vi "Reorient DH Matrix.vi"(10 "z":dbl[](array[numeric]), 11 "Original Frame":T1) -> (3 "Reoriented Frame":T1)   [LabVIEW 2017, in "NI_Robotics_3DKinematics.lvlib"]
uses:
  <vilib>/robotics/Kinematics/Plotting/NI_Robotics_3DKinematics.lvlib
  <vilib>/Analysis/Matrix/Datatypes/RealMatrix.ctl
  <vilib>/Analysis/_algsub.llb/Real Vector Norm.vi
  <vilib>/Analysis/NI_AALPro.lvlib
  <vilib>/robotics/Kinematics/NI_Kinematics.lvlib
  <vilib>/Analysis/Matrix/NI_Matrix.lvlib
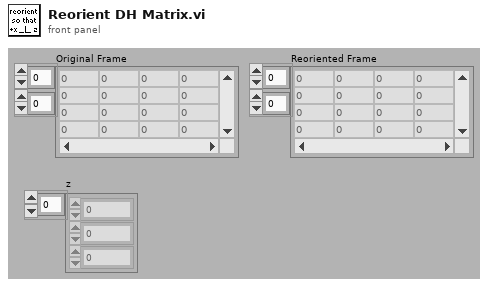
[diagram p1: front panel]
types:
  T1 = typedef "NI_Matrix.lvlib/RealMatrix.ctl" = dbl[][]
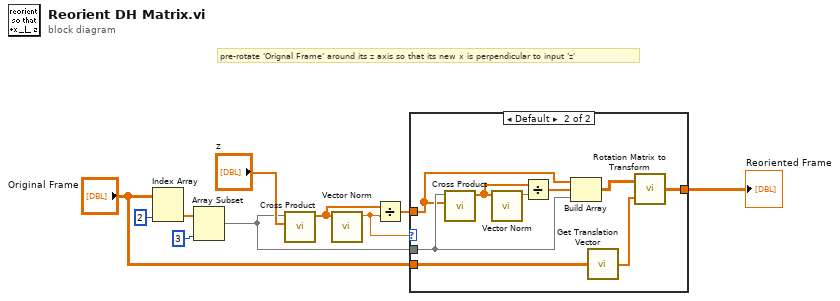
[diagram p0: block diagram]
diagram:
  # "pre-rotate 'Orignal Frame' around its z axis so that its new x is perpendicular to input 'z'"
  n1 = Index Array(array="Original Frame", index (col)=2 ("index (row)")) -> (element=w10:dbl[])  [unwired: 1 in]
  n2 = Array Subset(array=w10, length=3) -> (w1:dbl[])  [unwired: 1 in]
  n3 = call <vilib>:"Cross Product.vi"("B Vector"="z", "A Vector"=w1) -> ("Cross Product"=w4:dbl[])  [unwired: 8 in, 1 out]
  n4 = call-poly <vilib>:"Vector Norm.vi"("Input Vector"=w4) -> ("norm"=w5:dbl)  [unwired: 9 in, 1 out]
  n5 = Divide(x=w4, y=w5) -> (x/y=w6:dbl[])
  n6 = case shown="Default" w5 {
    tunnel: w6 -> [_ w14]
    tunnel: [w11 w15] -> w8
    tunnel: w1 -> [_ w16]
    tunnel: "Original Frame" -> [w11 w13]
    frame 0 {
    }
    frame Default {
      n7 = call <vilib>:"Cross Product.vi"("B Vector"=w14, "A Vector"=w16) -> ("Cross Product"=w19:dbl[])  [unwired: 8 in, 1 out]
      n8 = call-poly <vilib>:"Vector Norm.vi"("Input Vector"=w19) -> ("norm"=w20:dbl)  [unwired: 9 in, 1 out]
      n9 = Divide(x=w19, y=w20) -> (x/y=w18:dbl[])
      n10 = Build Array(w14, w18, w16) -> (w17:T1)
      n11 = call <vilib>:"Get Translation Vector.vi"("transform"=w13) -> ("translation vector"=w12:dbl[])
      n12 = call <vilib>:"Rotation Matrix to Transform.vi"("translation vector"=w12, "rotation matrix"=w17) -> ("transform"=w15:T1)
    }
  }
  "Reoriented Frame" <- w8
